vi "Initialize Protection Frames Incoming.vi"(8 "error in (no error)":errorcluster, 10 "Frames":T2[](array[typedef]) {"Protection Configurations"."CRC Channels"."Data Type" items=["Signed", "Unsigned", "IEEE Float"]}, 11 "PCL (usec)":u32) -> (0 "error out":errorcluster, 1 "Frame Values":T1, 2 "RT Frames":T9[](array[typedef]) {"Protection Configurations"."CRC Channels"."Data Type" items=["Signed", "Unsigned", "IEEE Float"]})   [LabVIEW 2019, in "Protection and Counter Support Engine.lvlib"]
uses:
  Protection and Counter Support Engine.lvlib
  Types/RT Frame Settings.ctl
  Shared/Types/Exported Frame Type.ctl
  Types/RT Protection Configuration.ctl
  Shared/Types/Protection Type.ctl
  Shared/Types/XNET Signal Configuration.ctl
  Shared/Types/Exported Counter Settings.ctl
  Shared/Types/Exported Event Trigger Type.ctl
  Shared/Types/Exported Frame Settings.ctl
  Shared/Types/Exported Protection Settings.ctl
  Types/RT Frame Incoming Values.ctl
  <vilib>/xnet/xnet.llb/XNET Create Session (Conversion).vi
  Shared/Protection and Counter Support Shared.lvlib
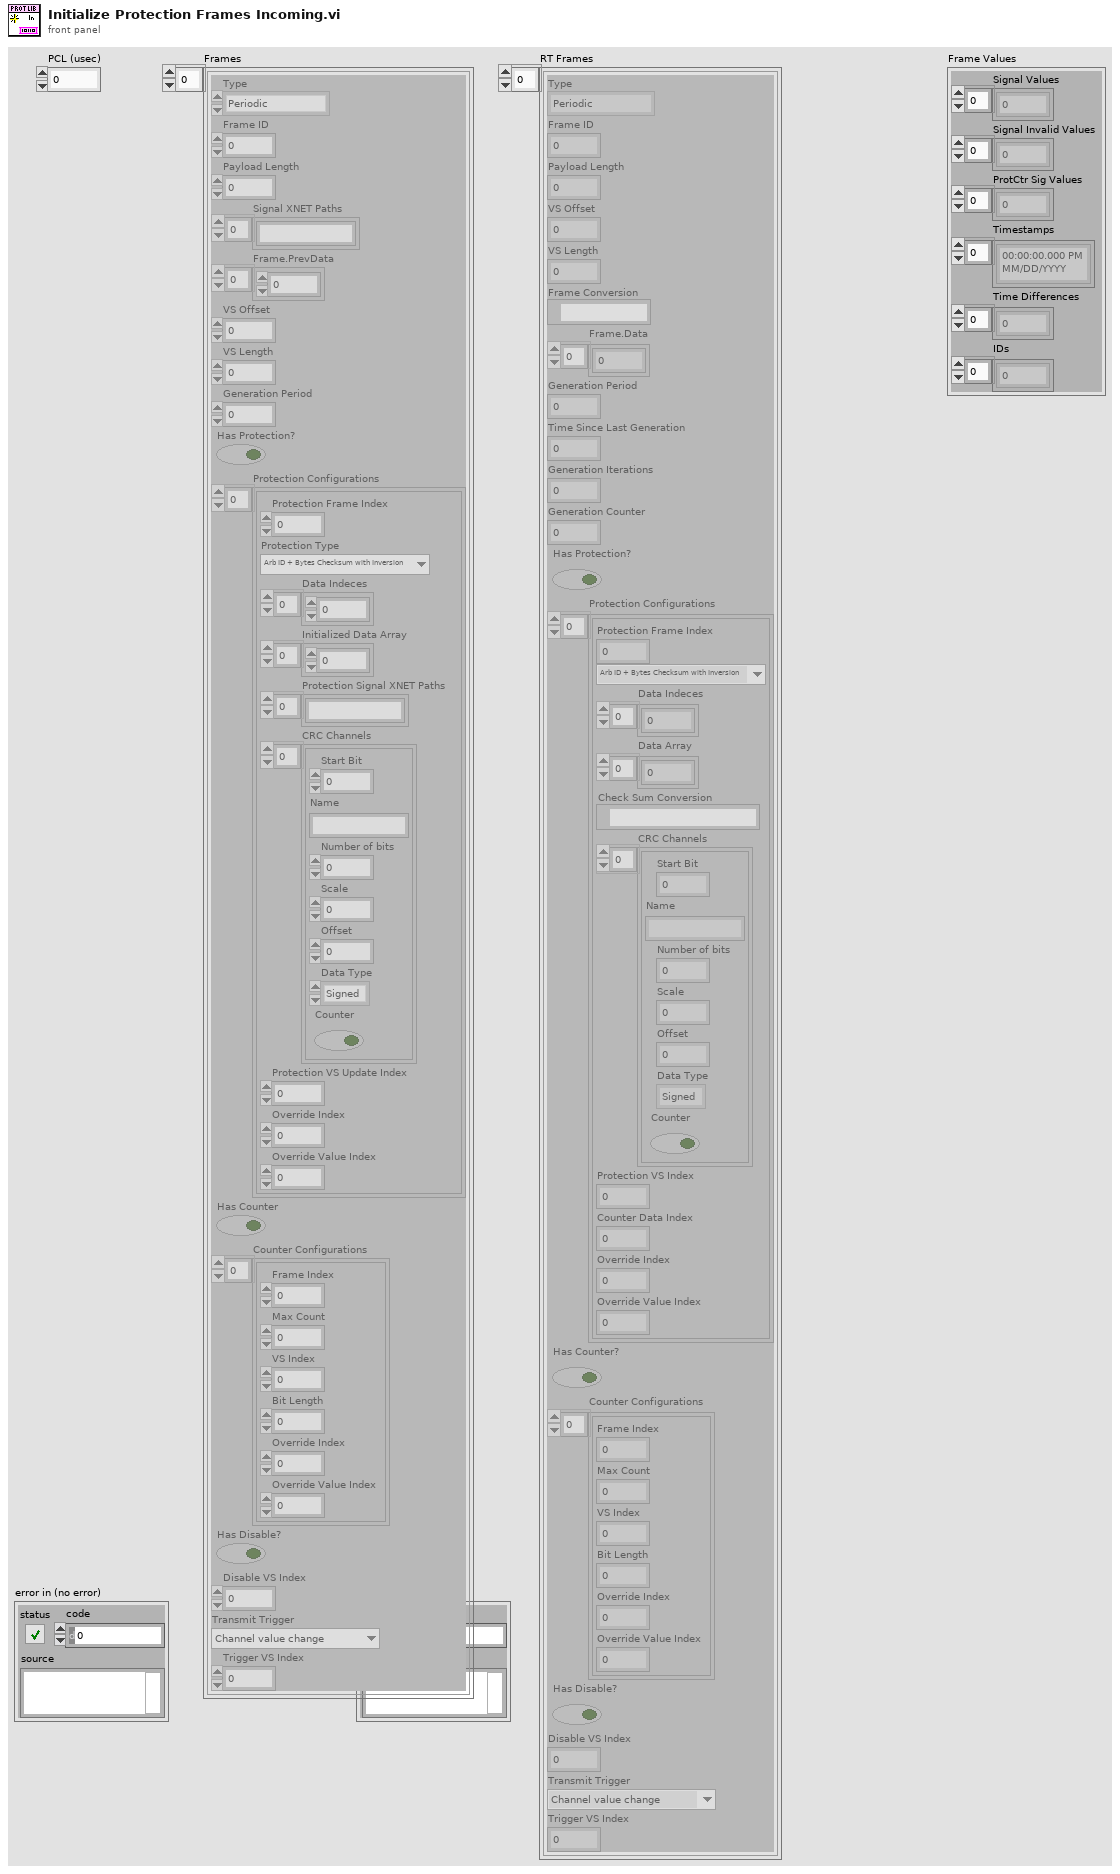
[diagram p1: front panel]
types:
  T1 = typedef "Protection and Counter Support Engine.lvlib/RT Frame Incoming Values.ctl" = cluster{"Signal Values":dbl[], "Signal Invalid Values":dbl[], "ProtCtr Sig Values":dbl[], "Timestamps":timestamp[], "Time Differences":dbl[], "IDs":u32[]}
  T2 = typedef "Protection and Counter Support Shared.lvlib/Exported Frame Settings.ctl" = cluster{"Type":T3, "Frame ID":u32, "Payload Length":u32, "Signal XNET Paths":string[], "Frame.PrevData":dbl[], "VS Offset":i32, "VS Length":i32, "Generation Period":u32, "Has Protection?":bool, "Protection Configurations":T4[], "Has Counter":bool, "Counter Configurations":T7[], "Has Disable?":bool, "Disable VS Index":i32, "Transmit Trigger":T8, "Trigger VS Index":i32}
  T3 = typedef "Protection and Counter Support Shared.lvlib/Exported Frame Type.ctl" = enum16{"Periodic", "Event", "Periodic/Event"}
  T4 = typedef "Protection and Counter Support Shared.lvlib/Exported Protection Settings.ctl" = cluster{"Protection Frame Index":i32, "Protection Type":T5, "Data Indeces":i32[], "Initialized Data Array":dbl[], "Protection Signal XNET Paths":string[], "CRC Channels":T6[], "Protection VS Update Index":i32, "Override Index":i32, "Override Value Index":i32}
  T5 = typedef "Protection and Counter Support Shared.lvlib/Protection Type.ctl" = enum16{"Arb ID + Bytes Checksum with Inversion", "Arb ID + Bytes CRC with Inversion", "Reversed Raw Signal Checksum with Inversion", "Concatenated Two's Compliment"}
  T6 = typedef "Protection and Counter Support Shared.lvlib/XNET Signal Configuration.ctl" = cluster{"Start Bit":i32, "Name":string, "Number of bits":i32, "Scale":dbl, "Offset":dbl, "Data Type":u32, "Counter":bool}
  T7 = typedef "Protection and Counter Support Shared.lvlib/Exported Counter Settings.ctl" = cluster{"Frame Index":i32, "Max Count":dbl, "VS Index":i32, "Bit Length":i64, "Override Index":i32, "Override Value Index":i32}
  T8 = typedef "Protection and Counter Support Shared.lvlib/Exported Event Trigger Type.ctl" = enum16{"Channel value change", "Trigger channel (not zero)", "Channel value change or trigger channel (not zero)", "Trigger channel (any value change)", "Channel value change or trigger channel (any value change)"}
  T9 = typedef "Protection and Counter Support Engine.lvlib/RT Frame Settings.ctl" = cluster{"Type":T3, "Frame ID":u32, "Payload Length":u32, "VS Offset":i32, "VS Length":i32, "Frame Conversion":refnum<k21>, "Frame.Data":dbl[], "Generation Period":u32, "Time Since Last Generation":u32, "Generation Iterations":u32, "Generation Counter":u32, "Has Protection?":bool, "Protection Configurations":T10[], "Has Counter?":bool, "Counter Configurations":T7[], "Has Disable?":bool, "Disable VS Index":i32, "Transmit Trigger":T8, "Trigger VS Index":i32}
  T10 = typedef "Protection and Counter Support Engine.lvlib/RT Protection Configuration.ctl" = cluster{"Protection Frame Index":i32, "Protection Type":T5, "Data Indeces":i32[], "Data Array":dbl[], "Check Sum Conversion":refnum<k21>, "CRC Channels":T6[], "Protection VS Index":i32, "Counter Data Index":i32, "Override Index":i32, "Override Value Index":i32}
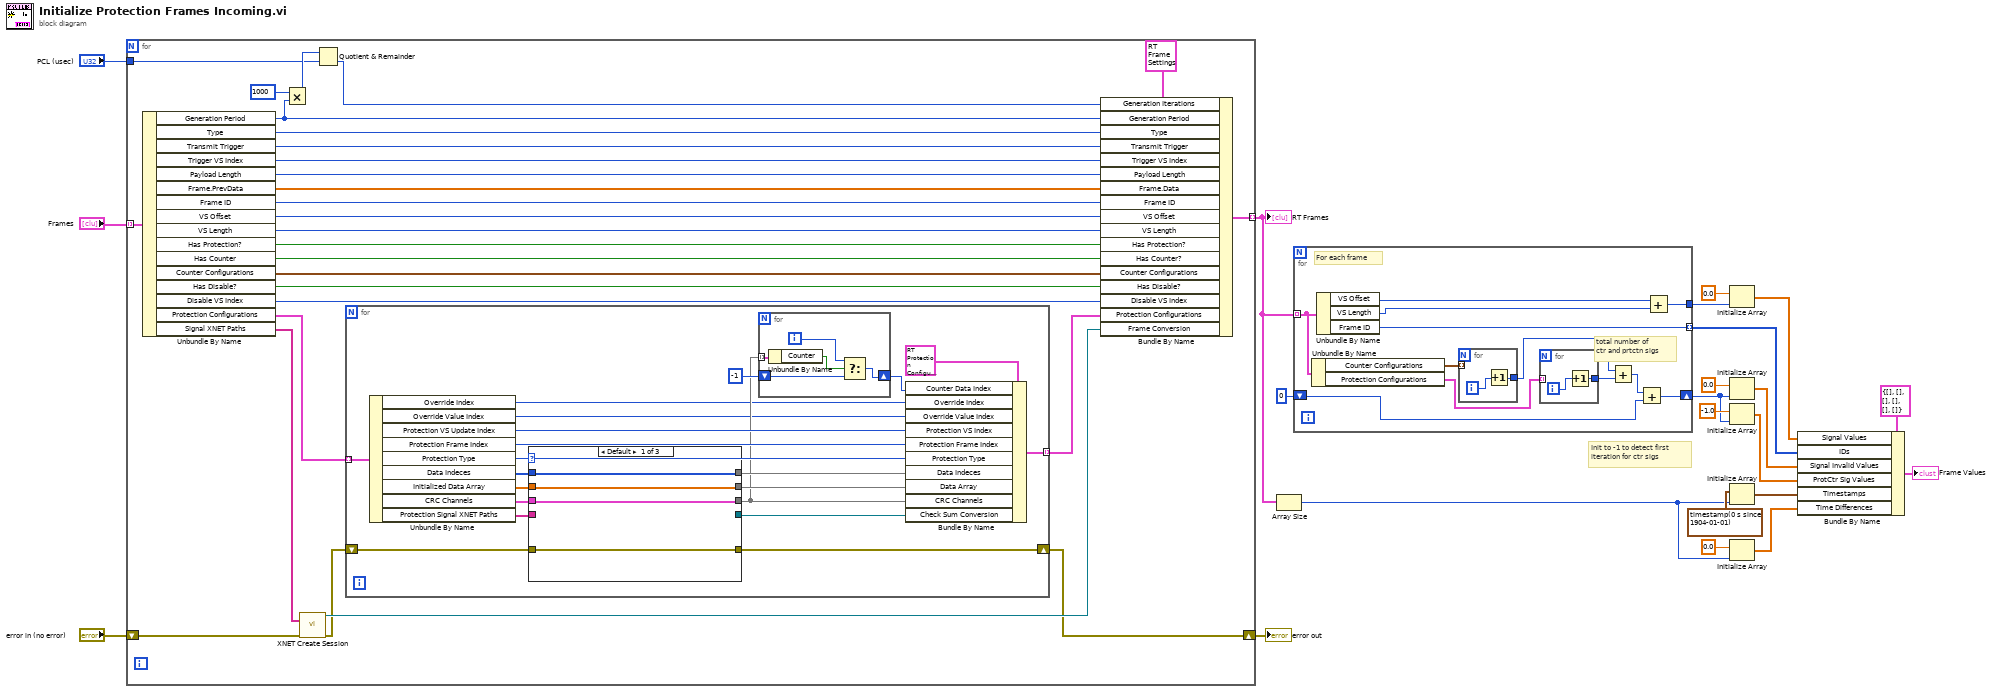
[diagram p0: block diagram]
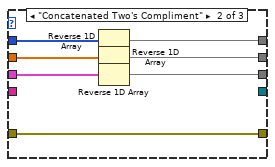
[diagram p2: hidden frame]
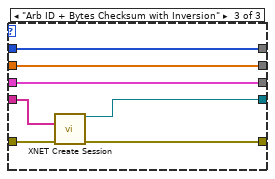
[diagram p3: hidden frame]
diagram:
  # "Init to -1 to detect first \niteration for ctr sigs"
  n1 = for {
    shift-right: [w35] -> w20
    shift-left: "error in (no error)" -> [w48]
    tunnel: "Frames" -> [w50] mode=indexing
    tunnel: [w34] -> w1 mode=indexing
    tunnel: "PCL (usec)" -> [w29]
    n2 = Unbundle By Name(w50) -> ("Generation Period"=w28:u32, "Type"=w23:T3, "Transmit Trigger"=w24:T8, "Trigger VS Index"=w25:i32, "Payload Length"=w26:u32, "Frame.PrevData"=w32:dbl[], "Frame ID"=w46:u32, "VS Offset"=w45:i32, "VS Length"=w44:i32, "Has Protection?"=w43:bool, "Has Counter"=w42:bool, "Counter Configurations"=w41:T7[], "Has Disable?"=w40:bool, "Disable VS Index"=w39:i32, "Protection Configurations"=w38:T4[], "Signal XNET Paths"=w49:string[])
    n3 = Multiply(x=u32 1000, y=w28) -> (x*y=w30:u32)
    n4 = call-poly <vilib>:"XNET Create Session.vi"("signal list"=w49, "error in (no error)"=w48) -> ("session out"=w47:refnum<k21>, "error out"=w36:errorcluster)  [unwired: 12 out]
    n5 = Quotient & Remainder(x=w30, y=w29) -> (floor(x/y)=w27:u32)  [unwired: 1 out]
    n6 = for {
      tunnel: w38 -> [w70] mode=indexing
      tunnel: [w65] -> w37 mode=indexing
      shift-right: [w63] -> w35
      shift-left: w36 -> [w64]
      n7 = Unbundle By Name(w70) -> ("Override Index"=w52:i32, "Override Value Index"=w51:i32, "Protection VS Update Index"=w54:i32, "Protection Frame Index"=w68:i32, "Protection Type"=w60:T5, "Data Indeces"=w55:i32[], "Initialized Data Array"=w57:dbl[], "CRC Channels"=w59:T6[], "Protection Signal XNET Paths"=w67:string[])
      n8 = case shown="Default" w60 {
        tunnel: w67 -> [_ _ w88]
        tunnel: [_ _ w87] -> w66
        tunnel: w64 -> [w74 w81 w86]
        tunnel: [w74 w81 w85] -> w63
        tunnel: [w73 w77 w84] -> w53
        tunnel: w59 -> [w73 w80 w84]
        tunnel: [w72 w76 w83] -> w58
        tunnel: w57 -> [w72 w79 w83]
        tunnel: [w71 w75 w82] -> w56
        tunnel: w55 -> [w71 w78 w82]
        frame Default {
        }
        frame "Concatenated Two's Compliment" {
          n9 = Reverse 1D Array(array=w78) -> (reversed array=w75:i32[])
          n10 = Reverse 1D Array(array=w79) -> (reversed array=w76:dbl[])
          n11 = Reverse 1D Array(array=w80) -> (reversed array=w77:T6[])
        }
        frame "Arb ID + Bytes Checksum with Inversion" {
          n12 = call-poly <vilib>:"XNET Create Session.vi"("signal list"=w88, "error in (no error)"=w86) -> ("session out"=w87:refnum<k21>, "error out"=w85:errorcluster)  [unwired: 12 out]
        }
      }
      n13 = for {
        tunnel: w53 -> [w93] mode=indexing
        shift-right: [w89] -> w61
        shift-left: -1 -> [w91]
        i -> [w90]
        n14 = Unbundle By Name(w93) -> ("Counter"=w92:bool)
        n15 = Select(t=w90, s=w92, f=w91) -> (s? t:f=w89:i32)
      }
      n16 = Bundle By Name(cluster=T10 {"Protection Frame Index"=0, "Protection Type"=enum."Arb ID + Bytes Checksum with Inversion", "Data Indeces"=[], "Data Array"=[], "Check Sum Conversion"="", "CRC Channels"=[], "Protection VS Index"=0, "Counter Data Index"=0, "Override Index"=0, "Override Value Index"=0} ("Cluster"), "Counter Data Index"=w61, "Override Index"=w52, "Override Value Index"=w51, "Protection VS Index"=w54, "Protection Frame Index"=w68, "Protection Type"=w60, "Data Indeces"=w56, "Data Array"=w58, "CRC Channels"=w53, "Check Sum Conversion"=w66) -> (w65:T10)
    }
    n17 = Bundle By Name(cluster=T9 {"Type"=enum."Periodic", "Frame ID"=0, "Payload Length"=0, "VS Offset"=0, "VS Length"=0, "Frame Conversion"="", "Frame.Data"=[], "Generation Period"=0, "Time Since Last Generation"=0, "Generation Iterations"=0, "Generation Counter"=0, "Has Protection?"=FALSE, "Protection Configurations"=[], "Has Counter?"=FALSE, "Counter Configurations"=[], "Has Disable?"=FALSE, "Disable VS Index"=0, "Transmit Trigger"=enum."Channel value change", "Trigger VS Index"=0} ("Frame Settings"), "Generation Iterations"=w27, "Generation Period"=w28, "Type"=w23, "Transmit Trigger"=w24, "Trigger VS Index"=w25, "Payload Length"=w26, "Frame.Data"=w32, "Frame ID"=w46, "VS Offset"=w45, "VS Length"=w44, "Has Protection?"=w43, "Has Counter?"=w42, "Counter Configurations"=w41, "Has Disable?"=w40, "Disable VS Index"=w39, "Protection Configurations"=w37, "Frame Conversion"=w47) -> (w34:T9)
  }
  "RT Frames" <- w1
  "error out" <- w20
  n18 = Array Size(array=w1) -> (size(s)=w6:i32)
  n19 = for {
    tunnel: w1 -> [w101] mode=indexing
    tunnel: [w105] -> w18 mode=indexing
    tunnel: [w102] -> w16
    shift-right: [w95] -> w12
    shift-left: 0 -> [w94]
    # "total number of\nctr and prtctn sigs"
    # "For each frame"
    n20 = Unbundle By Name(w101) -> ("Counter Configurations"=w100:T7[], "Protection Configurations"=w99:T10[])
    n21 = Unbundle By Name(w101) -> ("VS Offset"=w104:i32, "VS Length"=w103:i32, "Frame ID"=w105:u32)
    n22 = for {
      tunnel: w100 -> [_] mode=indexing
      tunnel: [w108] -> w98
      i -> [w109]
      n23 = Increment(x=w109) -> (x+1=w108:i32)
    }
    n24 = for {
      tunnel: [w106] -> w97
      tunnel: w99 -> [_] mode=indexing
      i -> [w107]
      n25 = Increment(x=w107) -> (x+1=w106:i32)
    }
    n26 = Add(x=w98, y=w97) -> (x+y=w96:i32)
    n27 = Add(x=w96, y=w94) -> (x+y=w95:i32)
    n28 = Add(x=w104, y=w103) -> (x+y=w102:i32)
  }
  n29 = Initialize Array(0.0, w16) -> (w15:dbl[])
  n30 = Initialize Array(0.0, w12) -> (w10:dbl[])
  n31 = Initialize Array(-1.0, w12) -> (w11:dbl[])
  n32 = Initialize Array(timestamp(0 s since 1904-01-01) ("Time Stamp"), w6) -> (w7:timestamp[])
  n33 = Initialize Array(0.0, w6) -> (w4:dbl[])
  n34 = Bundle By Name(cluster=T1 {"Signal Values"=[], "Signal Invalid Values"=[], "ProtCtr Sig Values"=[], "Timestamps"=[], "Time Differences"=[], "IDs"=[]} ("Incoming Values"), "Signal Values"=w15, "IDs"=w18, "Signal Invalid Values"=w10, "ProtCtr Sig Values"=w11, "Timestamps"=w7, "Time Differences"=w4) -> (→"Frame Values":T1)
